vi "TurretStateController.vi"(1 "Selected State (In)":string) -> (0 "Selected State (Out)":string)   [LabVIEW 2019]
uses:
  sensors.vi
  dsdata.vi
  outputs.vi
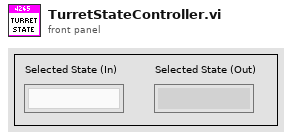
[diagram p1: front panel]
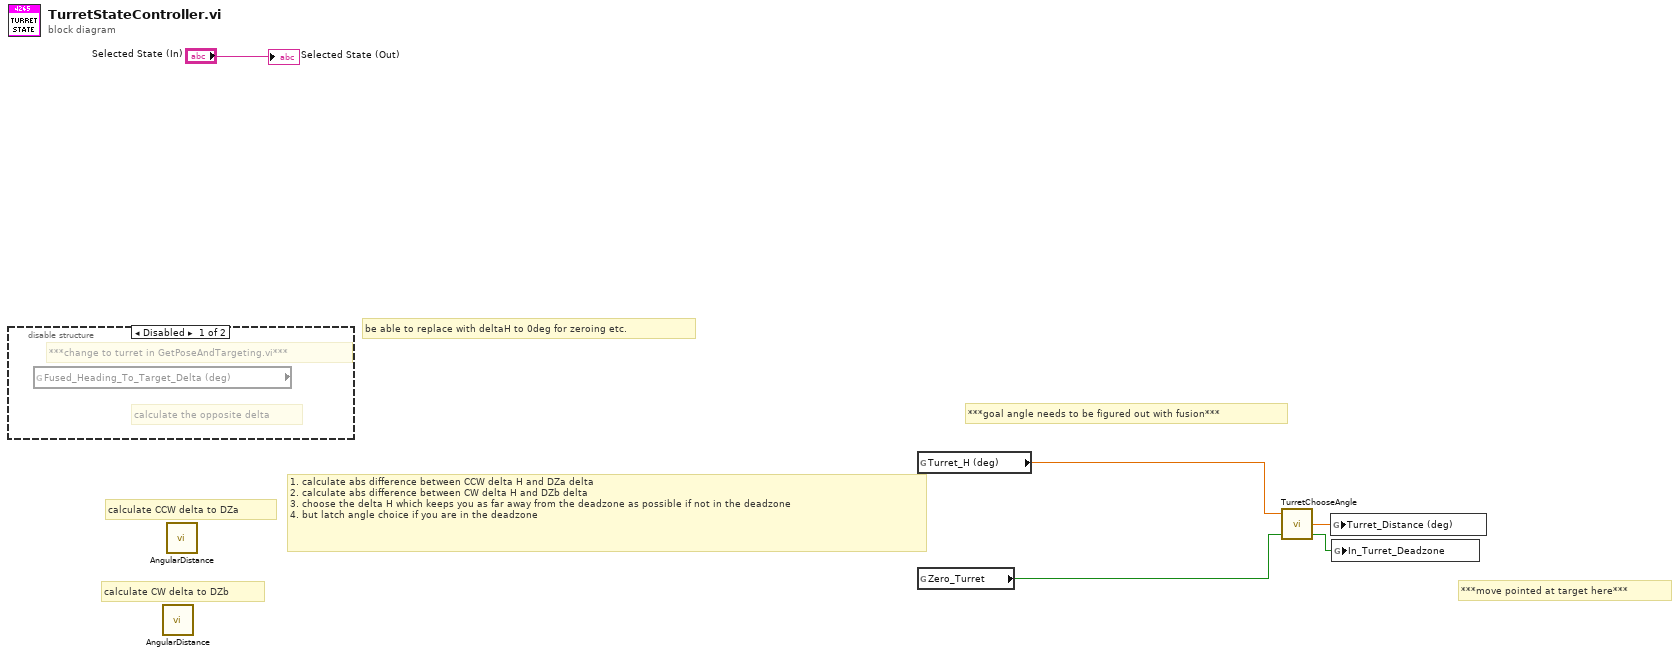
[diagram p0: block diagram]
diagram:
  # "be able to replace with deltaH to 0deg for zeroing etc."
  # "1. calculate abs difference between CCW delta H and DZa delta\n2. calculate abs difference between CW delta H and DZb delta\n3. choose the delta H which keeps you as far away from the deadzone as possible if not in the deadzone\n4. but latch angle choice if you are in the deadzone"
  # "calculate CW delta to DZb"
  # "calculate CCW delta to DZa"
  # "***goal angle needs to be figured out with fusion***"
  # "***move pointed at target here***"
  n1 = disable-structure shown="Disabled" {
    frame Disabled {
      # "calculate the opposite delta"
      # "***change to turret in GetPoseAndTargeting.vi***"
      n2 = global read "sensors.vi" "Fused_Heading_To_Target_Delta (deg)"() -> ()  [unwired: 1 out]
    }
    frame Enabled {
    }
  }
  n3 = call "AngularDistance.vi"() -> ()  [unwired: 2 in, 2 out]
  n4 = call "AngularDistance.vi"() -> ()  [unwired: 2 in, 2 out]
  n5 = global read "sensors.vi" "Turret_H (deg)"() -> (w4:dbl)
  n6 = global read "dsdata.vi" "Zero_Turret"() -> (w3:bool)
  n7 = call "TurretChooseAngle.vi"("Zero Turret"=w3, "Current Angle (deg)"=w4) -> ("In Deadzone"=w1:bool, "Angular Distance (deg)"=w2:dbl)  [unwired: 2 in]
  n8 = global write "outputs.vi" "Turret_Distance (deg)"(w2) -> ()
  n9 = global write "sensors.vi" "In_Turret_Deadzone"(w1) -> ()
  "Selected State (Out)" <- "Selected State (In)"
